vi "test_read-nmea-data2.vi"() -> ()   [LabVIEW 2019] (continued)
21,121,17,85,70,063,20,86,35,329,,3*73\n\t\n15:09:43.60\tF9P\t$GAGSV,2,1,08,02,09,298,16,04,66,119,29,09,31,193,22,11,71,357,23,7*77\n\t\n15:09:43.62\tF9P\t$GAGSV,2,2,08,12,40,102,19,19,27,045,15,25,10,250,,36,25,307,24,7*7E\n\t\n15:09:43.64\tF9P\t$GAGSV,2,1,08,02,09,298,,04,66,119,26,09,31,193,20,11,71,357,18,2*70\n\t\n15:09:43.66\tF9P\t$GAGSV,2,2,08,12,40,102,,19,27,045,,25,10,250,,36,25,307,30,2*72\n\t\n15:09:43.68\tF9P\t$GBGSV,1,1,03,11,51,130,38,14,86,148,29,33,59,218,27,1*47\n\t\n15:09:43.70\tF9P\t$GBGSV,1,1,04,08,,,20,11,51,130,23,14,86,148,26,33,59,218,,3*48\n\t\n15:09:43.72\tF9P\t$GNGLL,3723.59050,N,12656.89866,E,060945.00,A,A*7A\n\t\n15:09:43.74\tF9P\t\t\n15:09:43.76\tF9P\t\t\n15:09:43.78\tF9P\t\t\n15:09:43.80\tF9P\t\t\n15:09:43.82\tF9P\t\t\n15:09:43.84\tF9P\t\t\n15:09:43.86\tF9P\t\t\n15:09:43.88\tF9P\t\t\n15:09:43.90\tF9P\t\t\n15:09:43.92\tF9P\t\t\n15:09:43.94\tF9P\t\t\n15:09:43.96\tF9P\t\t\n15:09:43.98\tF9P\t\t\n15:09:44.00\tF9P\t\t\n15:09:44.02\tF9P\t\t\n15:09:44.04\tF9P\t\t\n15:09:44.06\tF9P\t\t\n15:09:44.08\tF9P\t\t\n15:09:44.10\tF9P\t\t\n15:09:44.12\tF9P\t\t\n15:09:44.14\tF9P\t\t\n15:09:44.16\tF9P\t\t\n15:09:44.18\tF9P\t\t\n15:09:44.20\tF9P\t\t\n15:09:44.22\tF9P\t\t\n15:09:44.24\tF9P\t\t\n15:09:44.26\tF9P\t$GNRMC,060946.00,A,3723.58981,N,12656.89795,E,2.353,239.48,250720,,,A,V*02\n\t\n15:09:44.28\tF9P\t$GNVTG,239.48,T,,M,2.353,N,4.358,K,A*2A\n\t\n15:09:44.30\tF9P\t$GNGGA,060946.00,3723.58981,N,12656.89795,E,1,12,0.75,42.1,M,18.5,M,,*71\n\t\n15:09:44.32\tF9P\t$GNGSA,A,3,12,06,19,05,17,09,04,02,,,,,1.51,0.75,1.31,1*04\n\t\n15:09:44.34\tF9P\t$GNGSA,A,3,85,71,84,,,,,,,,,,1.51,0.75,1.31,2*01\n\t\n15:09:44.36\tF9P\t$GNGSA,A,3,36,19,11,04,09,12,,,,,,,1.51,0.75,1.31,3*04\n\t\n15:09:44.38\tF9P\t$GNGSA,A,3,14,11,33,,,,,,,,,,1.51,0.75,1.31,4*05\n\t\n15:09:44.40\tF9P\t$GPGSV,3,1,09,02,54,318,33,04,19,044,23,05,36,246,27,06,65,046,35,1*6F\n\t\n15:09:44.42\tF9P\t$GPGSV,3,2,09,09,45,075,36,12,24,278,21,17,34,153,26,19,53,156,41,1*63\n\t\n15:09:44.44\tF9P\t$GPGSV,3,3,09,25,12,307,20,1*5F\n\t\n15:09:44.46\tF9P\t$GPGSV,3,1,09,02,54,318,,04,19,044,16,05,36,246,30,06,65,046,25,6*69\n\t\n15:09:44.48\tF9P\t$GPGSV,3,2,09,09,45,075,25,12,24,278,,17,34,153,15,19,53,156,,6*60\n\t\n15:09:44.50\tF9P\t$GPGSV,3,3,09,25,12,307,,6*5A\n\t\n15:09:44.52\tF9P\t$GLGSV,2,1,08,69,13,031,,70,73,042,,71,50,204,31,72,03,209,,1*73\n\t\n15:09:44.54\tF9P\t$GLGSV,2,2,08,77,01,327,,84,21,121,10,85,70,063,25,86,35,329,,1*73\n\t\n15:09:44.56\tF9P\t$GLGSV,2,1,08,69,13,031,11,70,73,042,,71,50,204,23,72,03,209,,3*72\n\t\n15:09:44.58\tF9P\t$GLGSV,2,2,08,77,01,327,,84,21,121,17,85,70,063,20,86,35,329,,3*73\n\t\n15:09:44.60\tF9P\t$GAGSV,2,1,08,02,09,298,16,04,66,119,29,09,31,193,23,11,71,357,22,7*77\n\t\n15:09:44.62\tF9P\t$GAGSV,2,2,08,12,40,102,19,19,27,045,13,25,10,250,,36,25,307,25,7*79\n\t\n15:09:44.64\tF9P\t$GAGSV,2,1,08,02,09,298,,04,66,119,26,09,31,193,21,11,71,357,17,2*7E\n\t\n15:09:44.66\tF9P\t$GAGSV,2,2,08,12,40,102,,19,27,045,,25,10,250,,36,25,307,22,2*71\n\t\n15:09:44.68\tF9P\t$GBGSV,1,1,03,11,51,130,33,14,86,148,29,33,59,218,28,1*43\n\t\n15:09:44.70\tF9P\t$GBGSV,1,1,04,08,,,21,11,51,130,23,14,86,148,24,33,59,218,,3*4B\n\t\n15:09:44.72\tF9P\t$GNGLL,3723.58981,N,12656.89795,E,060946.00,A,A*7E\n\t\n15:09:44.75\tF9P\t\t\n15:09:44.77\tF9P\t\t\n15:09:44.79\tF9P\t\t\n15:09:44.81\tF9P\t\t\n15:09:44.83\tF9P\t\t\n15:09:44.85\tF9P\t\t\n15:09:44.87\tF9P\t\t\n15:09:44.89\tF9P\t\t\n15:09:44.91\tF9P\t\t\n15:09:44.93\tF9P\t\t\n15:09:44.95\tF9P\t\t\n15:09:44.97\tF9P\t\t\n15:09:44.99\tF9P\t\t\n15:09:45.01\tF9P\t\t\n15:09:45.03\tF9P\t\t\n15:09:45.05\tF9P\t\t\n15:09:45.07\tF9P\t\t\n15:09:45.09\tF9P\t\t\n15:09:45.11\tF9P\t\t\n15:09:45.13\tF9P\t\t\n15:09:45.15\tF9P\t\t\n15:09:45.17\tF9P\t\t\n15:09:45.19\tF9P\t\t\n15:09:45.21\tF9P\t\t\n15:09:45.23\tF9P\t\t\n15:09:45.25\tF9P\t$GNRMC,060947.00,A,3723.58930,N,12656.89709,E,2.600,233.98,250720,,,A,V*08\n\t\n15:09:45.27\tF9P\t$GNVTG,233.98,T,,M,2.600,N,4.815,K,A*2C\n\t\n15:09:45.29\tF9P\t$GNGGA,060947.00,3723.58930,N,12656.89709,E,1,12,0.72,42.3,M,18.5,M,,*7A\n\t\n15:09:45.31\tF9P\t$GNGSA,A,3,12,06,19,05,17,09,04,02,,,,,1.36,0.72,1.16,1*07\n\t\n15:09:45.33\tF9P\t$GNGSA,A,3,85,71,84,,,,,,,,,,1.36,0.72,1.16,2*02\n\t\n15:09:45.35\tF9P\t$GNGSA,A,3,36,19,11,04,09,12,,,,,,,1.36,0.72,1.16,3*07\n\t\n15:09:45.37\tF9P\t$GNGSA,A,3,14,11,33,,,,,,,,,,1.36,0.72,1.16,4*06\n\t\n15:09:45.39\tF9P\t$GPGSV,3,1,09,02,54,318,29,04,19,044,21,05,36,246,26,06,65,046,32,1*60\n\t\n15:09:45.41\tF9P\t$GPGSV,3,2,09,09,45,075,27,12,24,278,22,17,34,153,24,19,53,156,32,1*66\n\t\n15:09:45.43\tF9P\t$GPGSV,3,3,09,25,12,307,20,1*5F\n\t\n15:09:45.45\tF9P\t$GPGSV,3,1,09,02,54,318,,04,19,044,16,05,36,246,29,06,65,046,25,6*61\n\t\n15:09:45.47\tF9P\t$GPGSV,3,2,09,09,45,075,23,12,24,278,,17,34,153,,19,53,156,,6*62\n\t\n15:09:45.49\tF9P\t$GPGSV,3,3,09,25,12,307,,6*5A\n\t\n15:09:45.51\tF9P\t$GLGSV,2,1,08,69,13,031,,70,73,042,,71,50,204,26,72,03,209,,1*75\n\t\n15:09:45.53\tF9P\t$GLGSV,2,2,08,77,01,327,,84,21,121,08,85,70,063,25,86,35,329,,1*7A\n\t\n15:09:45.55\tF9P\t$GLGSV,2,1,08,69,13,031,12,70,73,042,,71,50,204,22,72,03,209,,3*70\n\t\n15:09:45.57\tF9P\t$GLGSV,2,2,08,77,01,327,,84,21,121,17,85,70,063,21,86,35,329,,3*72\n\t\n15:09:45.59\tF9P\t$GAGSV,2,1,08,02,09,298,17,04,66,119,29,09,31,193,25,11,71,357,23,7*71\n\t\n15:09:45.61\tF9P\t$GAGSV,2,2,08,12,40,102,19,19,27,045,13,25,09,249,,36,25,307,27,7*7B\n\t\n15:09:45.63\tF9P\t$GAGSV,2,1,08,02,09,298,,04,66,119,24,09,31,193,21,11,71,357,16,2*7D\n\t\n15:09:45.65\tF9P\t$GAGSV,2,2,08,12,40,102,,19,27,045,,25,09,249,,36,25,307,23,2*70\n\t\n15:09:45.67\tF9P\t$GBGSV,1,1,03,11,51,130,36,14,86,148,28,33,59,218,27,1*48\n\t\n15:09:45.69\tF9P\t$GBGSV,1,1,04,08,,,21,11,51,130,24,14,86,148,23,33,59,218,,3*4B\n\t\n15:09:45.71\tF9P\t$GNGLL,3723.58930,N,12656.89709,E,060947.00,A,A*70\n\t\n15:09:45.73\tF9P\t\t\n15:09:45.75\tF9P\t\t\n15:09:45.77\tF9P\t\t\n15:09:45.79\tF9P\t\t\n15:09:45.81\tF9P\t\t\n15:09:45.83\tF9P\t\t\n15:09:45.85\tF9P\t\t\n15:09:45.87\tF9P\t\t\n15:09:45.89\tF9P\t\t\n15:09:45.91\tF9P\t\t\n15:09:45.93\tF9P\t\t\n15:09:45.95\tF9P\t\t\n15:09:45.97\tF9P\t\t\n15:09:45.99\tF9P\t\t\n15:09:46.01\tF9P\t\t\n15:09:46.03\tF9P\t\t\n15:09:46.05\tF9P\t\t\n15:09:46.07\tF9P\t\t\n15:09:46.09\tF9P\t\t\n15:09:46.11\tF9P\t\t\n15:09:46.13\tF9P\t\t\n15:09:46.15\tF9P\t\t\n15:09:46.17\tF9P\t\t\n15:09:46.19\tF9P\t\t\n15:09:46.21\tF9P\t\t\n15:09:46.23\tF9P\t\t\n15:09:46.25\tF9P\t$GNRMC,060948.00,A,3723.58899,N,12656.89591,E,2.440,246.59,250720,,,A,V*0F\n\t\n15:09:46.28\tF9P\t$GNVTG,246.59,T,,M,2.440,N,4.520,K,A*2E\n\t\n15:09:46.30\tF9P\t$GNGGA,060948.00,3723.58899,N,12656.89591,E,1,12,0.75,42.8,M,18.5,M,,*78\n\t\n15:09:46.32\tF9P\t$GNGSA,A,3,12,06,19,05,17,09,04,02,,,,,1.51,0.75,1.31,1*04\n\t\n15:09:46.34\tF9P\t$GNGSA,A,3,85,71,84,,,,,,,,,,1.51,0.75,1.31,2*01\n\t\n15:09:46.36\tF9P\t$GNGSA,A,3,36,19,11,04,09,12,,,,,,,1.51,0.75,1.31,3*04\n\t\n15:09:46.38\tF9P\t$GNGSA,A,3,14,11,33,,,,,,,,,,1.51,0.75,1.31,4*05\n\t\n15:09:46.40\tF9P\t$GPGSV,3,1,09,02,54,318,28,04,19,044,29,05,36,246,33,06,65,046,33,1*6C\n\t\n15:09:46.42\tF9P\t$GPGSV,3,2,09,09,45,075,33,12,24,278,21,17,34,153,23,19,53,156,37,1*62\n\t\n15:09:46.44\tF9P\t$GPGSV,3,3,09,25,12,307,21,1*5E\n\t\n15:09:46.46\tF9P\t$GPGSV,3,1,09,02,54,318,,04,19,044,16,05,36,246,30,06,65,046,25,6*69\n\t\n15:09:46.48\tF9P\t$GPGSV,3,2,09,09,45,075,23,12,24,278,,17,34,153,,19,53,156,,6*62\n\t\n15:09:46.50\tF9P\t$GPGSV,3,3,09,25,12,307,,6*5A\n\t\n15:09:46.52\tF9P\t$GLGSV,2,1,08,69,13,031,,70,73,042,,71,50,204,25,72,03,209,,1*76\n\t\n15:09:46.54\tF9P\t$GLGSV,2,2,08,77,01,327,,84,21,121,06,85,70,063,26,86,35,329,,1*77\n\t\n15:09:46.56\tF9P\t$GLGSV,2,1,08,69,13,031,13,70,73,042,,71,50,204,22,72,03,209,,3*71\n\t\n15:09:46.58\tF9P\t$GLGSV,2,2,08,77,01,327,,84,21,121,16,85,70,063,21,86,35,329,,3*73\n\t\n15:09:46.60\tF9P\t$GAGSV,2,1,08,02,09,298,16,04,66,119,28,09,31,193,25,11,71,357,25,7*77\n\t\n15:09:46.62\tF9P\t$GAGSV,2,2,08,12,40,102,19,19,27,045,12,25,09,249,,36,25,307,26,7*7B\n\t\n15:09:46.64\tF9P\t$GAGSV,2,1,08,02,09,298,,04,66,119,24,09,31,193,20,11,71,357,17,2*7D\n\t\n15:09:46.66\tF9P\t$GAGSV,2,2,08,12,40,102,,19,27,045,,25,09,249,,36,25,307,24,2*77\n\t\n15:09:46.68\tF9P\t$GBGSV,1,1,03,11,51,130,38,14,86,148,28,33,59,218,28,1*49\n\t\n15:09:46.70\tF9P\t$GBGSV,1,1,04,08,,,20,11,51,130,24,14,86,148,22,33,59,218,,3*4B\n\t\n15:09:46.72\tF9P\t$GNGLL,3723.58899,N,12656.89591,E,060948.00,A,A*7E\n\t\n15:09:46.74\tF9P\t\t\n15:09:46.76\tF9P\t\t\n15:09:46.78\tF9P\t\t\n15:09:46.80\tF9P\t\t\n15:09:46.82\tF9P\t\t\n15:09:46.84\tF9P\t\t\n15:09:46.86\tF9P\t\t\n15:09:46.88\tF9P\t\t\n15:09:46.90\tF9P\t\t\n15:09:46.92\tF9P\t\t\n15:09:46.94\tF9P\t\t\n15:09:46.96\tF9P\t\t\n15:09:46.98\tF9P\t\t\n15:09:47.00\tF9P\t\t\n15:09:47.02\tF9P\t\t\n15:09:47.04\tF9P\t\t\n15:09:47.06\tF9P\t\t\n15:09:47.08\tF9P\t\t\n15:09:47.10\tF9P\t\t\n15:09:47.12\tF9P\t\t\n15:09:47.14\tF9P\t\t\n15:09:47.16\tF9P\t\t\n15:09:47.18\tF9P\t\t\n15:09:47.20\tF9P\t\t\n15:09:47.22\tF9P\t\t\n15:09:47.24\tF9P\t\t\n15:09:47.26\tF9P\t$GNRMC,060949.00,A,3723.58869,N,12656.89512,E,1.649,248.30,250720,,,A,V*03\n\t\n15:09:47.28\tF9P\t$GNVTG,248.30,T,,M,1.649,N,3.054,K,A*26\n\t\n15:09:47.31\tF9P\t$GNGGA,060949.00,3723.58869,N,12656.89512,E,1,12,0.75,42.8,M,18.5,M,,*7D\n\t\n15:09:47.33\tF9P\t$GNGSA,A,3,12,06,19,05,17,09,04,02,,,,,1.51,0.75,1.31,1*04\n\t\n15:09:47.35\tF9P\t$GNGSA,A,3,85,71,84,,,,,,,,,,1.51,0.75,1.31,2*01\n\t\n15:09:47.37\tF9P\t$GNGSA,A,3,36,19,11,04,09,12,,,,,,,1.51,0.75,1.31,3*04\n\t\n15:09:47.39\tF9P\t$GNGSA,A,3,14,11,33,,,,,,,,,,1.51,0.75,1.31,4*05\n\t\n15:09:47.41\tF9P\t$GPGSV,3,1,09,02,54,318,36,04,19,044,21,05,36,246,29,06,65,046,36,1*65\n\t\n15:09:47.43\tF9P\t$GPGSV,3,2,09,09,45,075,28,12,24,278,21,17,34,153,21,19,53,156,38,1*65\n\t\n15:09:47.45\tF9P\t$GPGSV,3,3,09,25,12,307,21,1*5E\n\t\n15:09:47.47\tF9P\t$GPGSV,3,1,09,02,54,318,,04,19,044,14,05,36,246,29,06,65,046,25,6*63\n\t\n15:09:47.49\tF9P\t$GPGSV,3,2,09,09,45,075,21,12,24,278,,17,34,153,,19,53,156,,6*60\n\t\n15:09:47.51\tF9P\t$GPGSV,3,3,09,25,12,307,,6*5A\n\t\n15:09:47.53\tF9P\t$GLGSV,2,1,08,69,13,031,,70,73,042,,71,50,204,24,72,03,209,,1*77\n\t\n15:09:47.55\tF9P\t$GLGSV,2,2,08,77,01,327,,84,21,121,11,85,70,063,26,86,35,329,,1*71\n\t\n15:09:47.57\tF9P\t$GLGSV,2,1,08,69,13,031,13,70,73,042,,71,50,204,22,72,03,209,,3*71\n\t\n15:09:47.59\tF9P\t$GLGSV,2,2,08,77,01,327,,84,21,121,15,85,70,063,20,86,35,329,,3*71\n\t\n15:09:47.61\tF9P\t$GAGSV,2,1,08,02,09,298,13,04,66,119,29,09,31,193,24,11,71,357,25,7*72\n\t\n15:09:47.63\tF9P\t$GAGSV,2,2,08,12,40,102,17,19,27,045,11,25,09,249,,36,25,307,26,7*76\n\t\n15:09:47.65\tF9P\t$GAGSV,2,1,08,02,09,298,,04,66,119,24,09,31,193,20,11,71,357,18,2*72\n\t\n15:09:47.67\tF9P\t$GAGSV,2,2,08,12,40,102,,19,27,045,,25,09,249,,36,25,307,24,2*77\n\t\n15:09:47.69\tF9P\t$GBGSV,1,1,03,11,51,130,36,14,86,148,31,33,59,218,26,1*41\n\t\n15:09:47.71\tF9P\t$GBGSV,2,1,05,08,,,20,11,51,130,25,14,86,148,22,25,,,24,3*7E\n\t\n15:09:47.73\tF9P\t$GBGSV,2,2,05,33,59,218,,3*46\n\t\n15:09:47.75\tF9P\t$GNGLL,3723.58869,N,12656.89512,E,060949.00,A,A*7B\n\t\n15:09:47.77\tF9P\t\t\n15:09:47.79\tF9P\t\t\n15:09:47.81\tF9P\t\t\n15:09:47.83\tF9P\t\t\n15:09:47.85\tF9P\t\t\n15:09:47.87\tF9P\t\t\n15:09:47.89\tF9P\t\t\n15:09:47.91\tF9P\t\t\n15:09:47.93\tF9P\t\t\n15:09:47.95\tF9P\t\t\n15:09:47.97\tF9P\t\t\n15:09:47.99\tF9P\t\t\n15:09:48.01\tF9P\t\t\n15:09:48.03\tF9P\t\t\n15:09:48.05\tF9P\t\t\n15:09:48.07\tF9P\t\t\n15:09:48.09\tF9P\t\t\n15:09:48.11\tF9P\t\t\n15:09:48.13\tF9P\t\t\n15:09:48.15\tF9P\t\t\n15:09:48.17\tF9P\t\t\n15:09:48.19\tF9P\t\t\n15:09:48.21\tF9P\t\t\n15:09:48.23\tF9P\t\t\n15:09:48.25\tF9P\t$GNRMC,060950.00,A,3723.58816,N,12656.89403,E,2.118,243.29,250720,,,A,V*01\n\t\n15:09:48.27\tF9P\t$GNVTG,243.29,T,,M,2.118,N,3.923,K,A*2C\n\t\n15:09:48.29\tF9P\t$GNGGA,060950.00,3723.58816,N,12656.89403,E,1,12,0.72,43.6,M,18.5,M,,*74\n\t\n15:09:48.31\tF9P\t$GNGSA,A,3,12,06,19,05,17,09,04,02,,,,,1.36,0.72,1.16,1*07\n\t\n15:09:48.33\tF9P\t$GNGSA,A,3,85,71,84,,,,,,,,,,1.36,0.72,1.16,2*02\n\t\n15:09:48.35\tF9P\t$GNGSA,A,3,36,19,11,04,09,12,,,,,,,1.36,0.72,1.16,3*07\n\t\n15:09:48.37\tF9P\t$GNGSA,A,3,14,11,33,,,,,,,,,,1.36,0.72,1.16,4*06\n\t\n15:09:48.39\tF9P\t$GPGSV,3,1,09,02,54,318,30,04,19,044,19,05,36,246,30,06,65,046,35,1*63\n\t\n15:09:48.41\tF9P\t$GPGSV,3,2,09,09,45,075,28,12,24,278,20,17,34,153,21,19,53,156,42,1*69\n\t\n15:09:48.43\tF9P\t$GPGSV,3,3,09,25,12,307,22,1*5D\n\t\n15:09:48.45\tF9P\t$GPGSV,3,1,09,02,54,318,,04,19,044,11,05,36,246,30,06,65,046,26,6*6D\n\t\n15:09:48.47\tF9P\t$GPGSV,3,2,09,09,45,075,22,12,24,278,,17,34,153,,19,53,156,,6*63\n\t\n15:09:48.49\tF9P\t$GPGSV,3,3,09,25,12,307,,6*5A\n\t\n15:09:48.51\tF9P\t$GLGSV,2,1,08,69,13,031,,70,73,042,,71,50,204,25,72,03,209,,1*76\n\t\n15:09:48.53\tF9P\t$GLGSV,2,2,08,77,01,327,,84,21,121,11,85,70,063,25,86,35,329,,1*72\n\t\n15:09:48.55\tF9P\t$GLGSV,2,1,08,69,13,031,14,70,73,042,,71,50,204,20,72,03,209,,3*74\n\t\n15:09:48.57\tF9P\t$GLGSV,2,2,08,77,01,327,,84,21,121,11,85,70,063,19,86,35,329,,3*7F\n\t\n15:09:48.59\tF9P\t$GAGSV,2,1,08,02,09,298,15,04,66,119,33,09,31,193,25,11,71,357,24,7*7F\n\t\n15:09:48.61\tF9P\t$GAGSV,2,2,08,12,40,102,18,19,27,045,09,25,09,249,,36,25,307,26,7*70\n\t\n15:09:48.63\tF9P\t$GAGSV,2,1,08,02,09,298,,04,66,119,26,09,31,193,20,11,71,357,17,2*7F\n\t\n15:09:48.65\tF9P\t$GAGSV,2,2,08,12,40,102,,19,27,045,,25,09,249,,36,25,307,23,2*70\n\t\n15:09:48.67\tF9P\t$GBGSV,1,1,03,11,51,130,41,14,86,148,32,33,59,218,26,1*42\n\t\n15:09:48.69\tF9P\t$GBGSV,1,1,04,08,,,19,11,51,130,25,14,86,148,23,33,59,218,,3*41\n\t\n15:09:48.71\tF9P\t$GNGLL,3723.58816,N,12656.89403,E,060950.00,A,A*7A\n\t\n15:09:48.73\tF9P\t\t\n15:09:48.75\tF9P\t\t\n15:09:48.77\tF9P\t\t\n15:09:48.79\tF9P\t\t\n15:09:48.81\tF9P\t\t\n15:09:48.83\tF9P\t\t\n15:09:48.85\tF9P\t\t\n15:09:48.87\tF9P\t\t\n15:09:48.89\tF9P\t\t\n15:09:48.91\tF9P\t\t\n15:09:48.93\tF9P\t\t\n15:09:48.95\tF9P\t\t\n15:09:48.97\tF9P\t\t\n15:09:48.99\tF9P\t\t\n15:09:49.01\tF9P\t\t\n15:09:49.03\tF9P\t\t\n15:09:49.05\tF9P\t\t\n15:09:49.07\tF9P\t\t\n15:09:49.09\tF9P\t\t\n15:09:49.11\tF9P\t\t\n15:09:49.13\tF9P\t\t\n15:09:49.15\tF9P\t\t\n15:09:49.17\tF9P\t\t\n15:09:49.19\tF9P\t\t\n15:09:49.21\tF9P\t\t\n15:09:49.23\tF9P\t\t\n15:09:49.25\tF9P\t$GNRMC,060951.00,A,3723.58776,N,12656.89324,E,2.472,238.67,250720,,,A,V*04\n\t\n15:09:49.27\tF9P\t$GNVTG,238.67,T,,M,2.472,N,4.578,K,A*26\n\t\n15:09:49.29\tF9P\t$GNGGA,060951.00,3723.58776,N,12656.89324,E,1,12,0.72,43.1,M,18.5,M,,*79\n\t\n15:09:49.31\tF9P\t$GNGSA,A,3,12,06,19,05,17,09,02,,,,,,1.36,0.72,1.16,1*03\n\t\n15:09:49.33\tF9P\t$GNGSA,A,3,85,71,84,,,,,,,,,,1.36,0.72,1.16,2*02\n\t\n15:09:49.35\tF9P\t$GNGSA,A,3,36,19,11,04,09,12,,,,,,,1.36,0.72,1.16,3*07\n\t\n15:09:49.37\tF9P\t$GNGSA,A,3,14,11,33,,,,,,,,,,1.36,0.72,1.16,4*06\n\t\n15:09:49.39\tF9P\t$GPGSV,3,1,09,02,54,318,29,04,19,044,17,05,36,246,34,06,65,046,32,1*66\n\t\n15:09:49.41\tF9P\t$GPGSV,3,2,09,09,45,075,22,12,24,278,20,17,34,153,21,19,53,156,34,1*62\n\t\n15:09:49.43\tF9P\t$GPGSV,3,3,09,25,12,307,21,1*5E\n\t\n15:09:49.45\tF9P\t$GPGSV,3,1,09,02,54,318,,04,19,044,,05,36,246,29,06,65,046,26,6*65\n\t\n15:09:49.47\tF9P\t$GPGSV,3,2,09,09,45,075,22,12,24,278,,17,34,153,,19,53,156,,6*63\n\t\n15:09:49.49\tF9P\t$GPGSV,3,3,09,25,12,307,,6*5A\n\t\n15:09:49.51\tF9P\t$GLGSV,2,1,08,69,13,031,,70,73,042,,71,50,204,25,72,03,209,,1*76\n\t\n15:09:49.53\tF9P\t$GLGSV,2,2,08,77,01,327,,84,21,121,09,85,70,063,24,86,35,329,,1*7A\n\t\n15:09:49.55\tF9P\t$GLGSV,2,1,08,69,13,031,11,70,73,042,,71,50,204,20,72,03,209,,3*71\n\t\n15:09:49.57\tF9P\t$GLGSV,2,2,08,77,01,327,,84,21,121,10,85,70,063,20,86,35,329,,3*74\n\t\n15:09:49.59\tF9P\t$GAGSV,2,1,08,02,09,298,16,04,66,119,32,09,31,193,25,11,71,357,31,7*79\n\t\n15:09:49.61\tF9P\t$GAGSV,2,2,08,12,40,102,18,19,27,045,11,25,09,249,,36,25,307,26,7*79\n\t\n15:09:49.63\tF9P\t$GAGSV,2,1,08,02,09,298,,04,66,119,25,09,31,193,19,11,71,357,18,2*79\n\t\n15:09:49.65\tF9P\t$GAGSV,2,2,08,12,40,102,,19,27,045,,25,09,249,,36,25,307,30,2*72\n\t\n15:09:49.67\tF9P\t$GBGSV,1,1,03,11,51,130,34,14,86,148,28,33,59,218,26,1*4B\n\t\n15:09:49.69\tF9P\t$GBGSV,1,1,04,08,,,20,11,51,130,25,14,86,148,22,33,59,218,,3*4A\n\t\n15:09:49.71\tF9P\t$GNGLL,3723.58776,N,12656.89324,E,060951.00,A,A*70\n\t\n15:09:49.73\tF9P\t\t\n15:09:49.75\tF9P\t\t\n15:09:49.77\tF9P\t\t\n15:09:49.79\tF9P\t\t\n15:09:49.81\tF9P\t\t\n15:09:49.83\tF9P\t\t\n15:09:49.85\tF9P\t\t\n15:09:49.87\tF9P\t\t\n15:09:49.89\tF9P\t\t\n15:09:49.91\tF9P\t\t\n15:09:49.93\tF9P\t\t\n15:09:49.95\tF9P\t\t\n15:09:49.97\tF9P\t\t\n15:09:49.99\tF9P\t\t\n15:09:50.01\tF9P\t\t\n15:09:50.03\tF9P\t\t\n15:09:50.05\tF9P\t\t\n15:09:50.07\tF9P\t\t\n15:09:50.09\tF9P\t\t\n15:09:50.11\tF9P\t\t\n15:09:50.13\tF9P\t\t\n15:09:50.15\tF9P\t\t\n15:09:50.17\tF9P\t\t\n15:09:50.19\tF9P\t\t\n15:09:50.21\tF9P\t\t\n15:09:50.23\tF9P\t\t\n15:09:50.25\tF9P\t$GNRMC,060952.00,A,3723.58757,N,12656.89187,E,1.579,245.30,250720,,,A,V*0E\n\t\n15:09:50.27\tF9P\t$GNVTG,245.30,T,,M,1.579,N,2.924,K,A*24\n\t\n15:09:50.29\tF9P\t$GNGGA,060952.00,3723.58757,N,12656.89187,E,1,12,0.75,42.6,M,18.5,M,,*73\n\t\n15:09:50.31\tF9P\t$GNGSA,A,3,12,06,19,05,17,09,04,02,,,,,1.51,0.75,1.31,1*04\n\t\n15:09:50.33\tF9P\t$GNGSA,A,3,85,71,,,,,,,,,,,1.51,0.75,1.31,2*0D\n\t\n15:09:50.35\tF9P\t$GNGSA,A,3,36,19,11,04,09,12,,,,,,,1.51,0.75,1.31,3*04\n\t\n15:09:50.37\tF9P\t$GNGSA,A,3,14,11,33,,,,,,,,,,1.51,0.75,1.31,4*05\n\t\n15:09:50.39\tF9P\t$GPGSV,3,1,09,02,54,318,24,04,19,044,15,05,36,246,38,06,65,046,35,1*62\n\t\n15:09:50.41\tF9P\t$GPGSV,3,2,09,09,45,075,21,12,24,278,18,17,34,153,20,19,53,156,29,1*67\n\t\n15:09:50.43\tF9P\t$GPGSV,3,3,09,25,12,307,20,1*5F\n\t\n15:09:50.45\tF9P\t$GPGSV,3,1,09,02,54,318,,04,19,044,,05,36,246,21,06,65,046,24,6*6F\n\t\n15:09:50.47\tF9P\t$GPGSV,3,2,09,09,45,075,21,12,24,278,,17,34,153,,19,53,156,,6*60\n\t\n15:09:50.49\tF9P\t$GPGSV,3,3,09,25,12,307,,6*5A\n\t\n15:09:50.51\tF9P\t$GLGSV,2,1,08,69,13,031,,70,73,042,,71,50,204,27,72,03,209,,1*74\n\t\n15:09:50.53\tF9P\t$GLGSV,2,2,08,77,01,327,,84,21,121,07,85,70,063,24,86,35,329,,1*74\n\t\n15:09:50.55\tF9P\t$GLGSV,2,1,08,69,13,031,,70,73,042,,71,50,204,21,72,03,209,,3*70\n\t\n15:09:50.57\tF9P\t$GLGSV,2,2,08,77,01,327,,84,21,121,09,85,70,063,18,86,35,329,,3*77\n\t\n15:09:50.59\tF9P\t$GAGSV,2,1,08,02,09,298,,04,66,119,26,09,31,193,30,11,71,357,24,7*7B\n\t\n15:09:50.61\tF9P\t$GAGSV,2,2,08,12,40,102,19,19,27,045,11,25,09,249,,36,25,307,25,7*7B\n\t\n15:09:50.63\tF9P\t$GAGSV,2,1,08,02,09,298,,04,66,119,23,09,31,193,21,11,71,357,19,2*75\n\t\n15:09:50.65\tF9P\t$GAGSV,2,2,08,12,40,102,,19,27,045,,25,09,249,,36,25,307,,2*71\n\t\n15:09:50.67\tF9P\t$GBGSV,1,1,03,11,51,130,35,14,86,148,21,33,59,218,26,1*43\n\t\n15:09:50.69\tF9P\t$GBGSV,1,1,04,08,,,21,11,51,130,25,14,86,148,21,33,59,218,,3*48\n\t\n15:09:50.71\tF9P\t$GNGLL,3723.58757,N,12656.89187,E,060952.00,A,A*7B\n\t\n15:09:50.73\tF9P\t\t\n15:09:50.75\tF9P\t\t\n15:09:50.77\tF9P\t\t\n15:09:50.79\tF9P\t\t\n15:09:50.81\tF9P\t\t\n15:09:50.83\tF9P\t\t\n15:09:50.85\tF9P\t\t\n15:09:50.87\tF9P\t\t\n15:09:50.89\tF9P\t\t\n15:09:50.91\tF9P\t\t\n15:09:50.93\tF9P\t\t\n15:09:50.95\tF9P\t\t\n15:09:50.97\tF9P\t\t\n15:09:50.99\tF9P\t\t\n15:09:51.01\tF9P\t\t\n15:09:51.03\tF9P\t\t\n15:09:51.05\tF9P\t\t\n15:09:51.07\tF9P\t\t\n15:09:51.09\tF9P\t\t\n15:09:51.11\tF9P\t\t\n15:09:51.13\tF9P\t\t\n15:09:51.15\tF9P\t\t\n15:09:51.17\tF9P\t\t\n15:09:51.19\tF9P\t\t\n15:09:51.21\tF9P\t\t\n15:09:51.23\tF9P\t\t\n15:09:51.25\tF9P\t$GNRMC,060953.00,A,3723.58734,N,12656.89105,E,1.629,246.51,250720,,,A,V*02\n\t\n15:09:51.27\tF9P\t$GNVTG,246.51,T,,M,1.629,N,3.017,K,A*2E\n\t\n15:09:51.29\tF9P\t$GNGGA,060953.00,3723.58734,N,12656.89105,E,1,12,0.72,41.9,M,18.5,M,,*76\n\t\n15:09:51.31\tF9P\t$GNGSA,A,3,12,06,19,05,17,09,02,,,,,,1.36,0.72,1.16,1*03\n\t\n15:09:51.33\tF9P\t$GNGSA,A,3,85,71,84,,,,,,,,,,1.36,0.72,1.16,2*02\n\t\n15:09:51.35\tF9P\t$GNGSA,A,3,36,19,11,04,09,12,,,,,,,1.36,0.72,1.16,3*07\n\t\n15:09:51.37\tF9P\t$GNGSA,A,3,14,11,33,,,,,,,,,,1.36,0.72,1.16,4*06\n\t\n15:09:51.39\tF9P\t$GPGSV,3,1,09,02,54,318,35,04,19,044,,05,36,246,36,06,65,046,27,1*6B\n\t\n15:09:51.41\tF9P\t$GPGSV,3,2,09,09,45,075,29,12,24,278,19,17,34,153,18,19,53,156,36,1*6B\n\t\n15:09:51.43\tF9P\t$GPGSV,3,3,09,25
